vi "Global Variables.vi"() -> ()   [LabVIEW 2011]
panel:
  in  "Disable GPS VISA":bool
  in  "GPS Data":T1={"GPS VISA resource name"="COM3", "GPS Error"={"status"=FALSE, "code"=0, "source"=""}}
  in  "Initial Encoder Counts":string="0" caption="Enter number in encoder counts, 0 is middle, -650000 fully entended; 650000 fully retracted"
  in  "Disable XBox Drive & Steer":bool
  in  "# of Parallel Routes":u32=4
  in  "Turn Right Encoder Counts [0-(-500000) Counts]":string="-500000"
  in  "Turn Left Encoder Counts [0-500000 Counts]":string="500000"
  in  "Stop Duration [0-4000 Milliseconds]":u32=2000
  in  "Turn Duration [0-10000 Milliseconds]":u32=6000
  in  "Turn Speed [0-5 Volts]":string="1"
  in  "Drive Duration [0-10000 Milliseconds]":u32=4000
  in  "Drive Speed [0-5 Volts]":string="3"
  in  "Button B":bool
  in  "Button A":bool
  out "Galil Data":T2
  out "Xbox Data":T3
  in  "End Program":bool
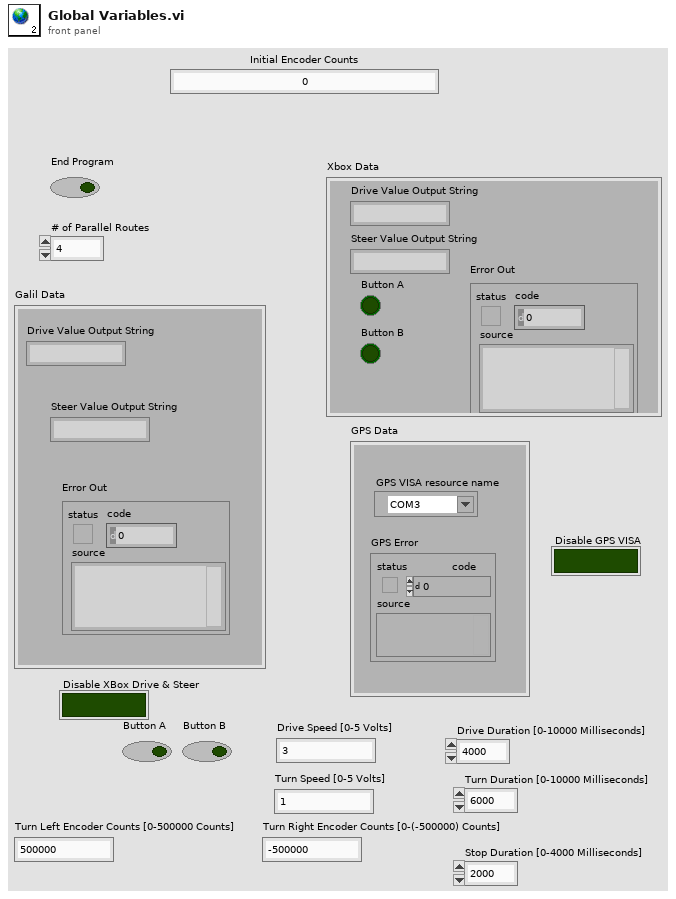
[diagram p1: front panel]
types:
  T1 = cluster{"GPS VISA resource name":refnum<visa-resource-name>, "GPS Error":errorcluster}
  T2 = cluster{"Drive Value Output String":string, "Steer Value Output String":string, "Error Out":errorcluster}
  T3 = cluster{"Drive Value Output String":string, "Steer Value Output String":string, "Button A":bool, "Button B":bool, "Error Out":errorcluster}
diagram:
